vi "IDN.vi"(8 "error in (no error)":errorcluster, 9 "Low module address":i32=120, 10 "High module address":i32=123, 11 "RP Communicator in":refnum<class "RP Communicator.lvclass">) -> (0 "error out":errorcluster, 1 "Logic tag":u16, 2 "IDN response":u32=1 format="0x%x (%d)", 3 "RP Communicator out":refnum<class "RP Communicator.lvclass">, 4 "Status response":u32=1 format="0x%x (%d)", 5 "DDS modulus":i64, 6 "Module":i32)   [LabVIEW 2024, in "RP Communicator.lvclass"]
uses:
  RP Communicator.lvclass
  RP Communicator.lvclass/RP Communicator.ctl
  RP Command.ctl
  RP Write Command TCP.vi
  RP Read Status TCP.vi
  RP Status Offsets.ctl
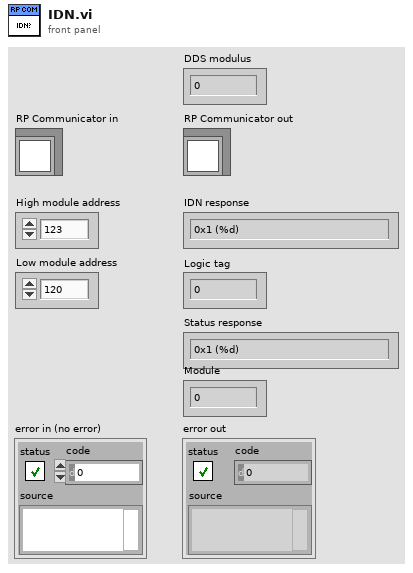
[diagram p1: front panel]
types:
  T1 = typedef "RP Command.ctl" = enum16{"Reset", "Read IDN", "Stop server", "Get status", "Get temperature", "Connect client", "Arm", "Software trigger", "Get whole buffer", "Get chunk", "System call", "Get config", "Set config", "Recieve data", "Recieve Calibartion", "Transmit data"}
  T2 = enum16{"big-endian, network order", "native, host order", "little-endian"}
  T3 = typedef "RP Status Offsets.ctl" = u16
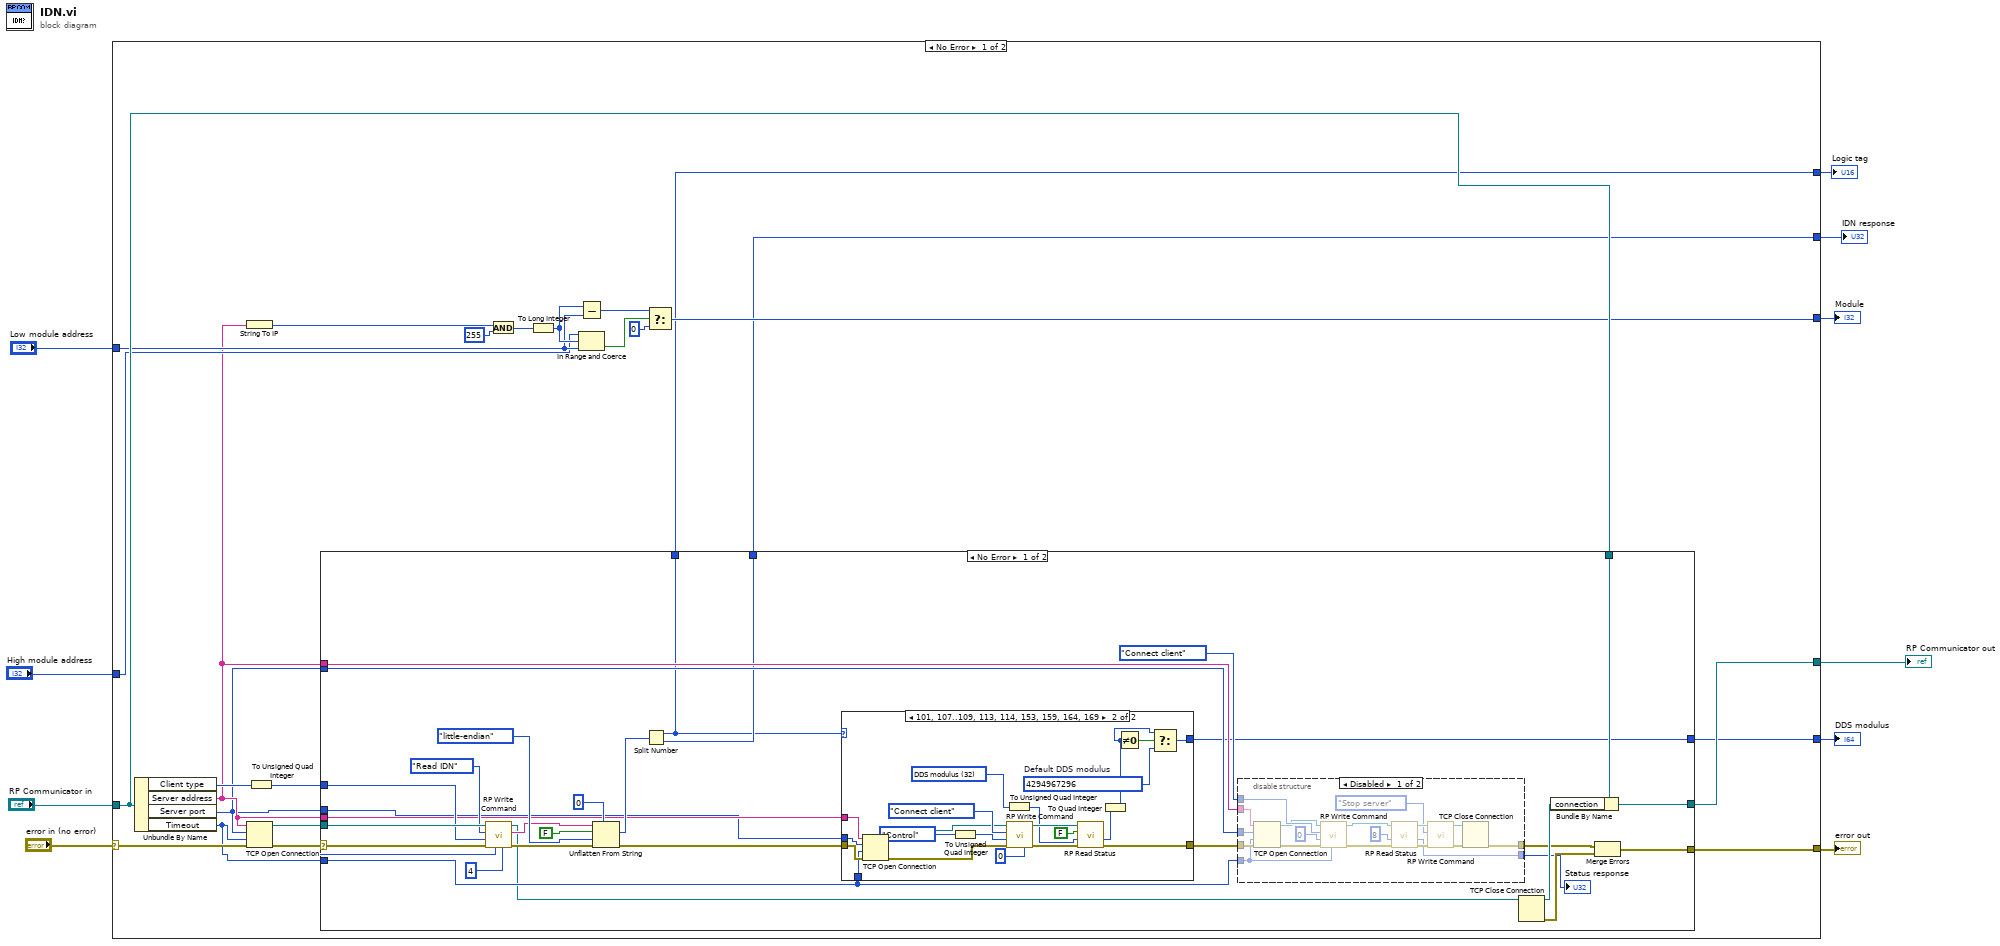
[diagram p0: block diagram]
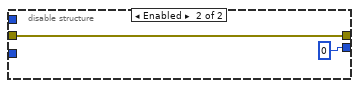
[diagram p3: hidden frame]
diagram:
  n1 = case shown="No Error" "error in (no error)" {
    selector: "error in (no error)" -> [w34 w110]
    tunnel: [w28 w110] -> w9
    tunnel: [w30 w109] -> w7
    tunnel: "RP Communicator in" -> [w31 w109]
    tunnel: [w17 _] -> w6
    tunnel: "Low module address" -> [w22 _]
    tunnel: "High module address" -> [w21 _]
    tunnel: [w16 _] -> w3
    tunnel: [w15 _] -> w2
    tunnel: [w14 _] -> w1
    frame No Error {
      n2 = Unbundle By Name(w31) -> ("Client type"=w32:enum16{"Control", "Reciever", "Transmitter"}, "Server address"=w12:string, "Server port"=w11:u16, "Timeout"=w27:i32)
      n3 = String To IP(1:w12) -> (0:w26:u32)
      n4 = TCP Open Connection(address=w12, remote port or service name=w11, timeout ms (60000)=w27, error in (no error)=w34) -> (connection ID=w33:refnum<k5>, error out=w13:errorcluster)  [unwired: 1 in]
      n5 = To Unsigned Quad Integer(1:w32) -> (0:w29:u64)
      n6 = case shown="No Error" w13 {
        selector: w13 -> [w39 w108]
        tunnel: w33 -> [w64 _]
        tunnel: w31 -> [w63 w107]
        tunnel: [w62 w107] -> w30
        tunnel: w29 -> [w60 _]
        tunnel: [w54 w108] -> w28
        tunnel: w11 -> [w50 _]
        tunnel: w27 -> [w36 _]
        tunnel: w12 -> [w48 _]
        tunnel: [w45 _] -> w16
        tunnel: [w41 _] -> w15
        tunnel: [w40 _] -> w14
        tunnel: w12 -> [w38 _]
        tunnel: w11 -> [w37 _]
        frame No Error {
          n7 = call-poly "RP Write Command.vi"("bytes to read"=4, "timeout ms (25000)"=w36, "Error In"=w39, "Command payload"=w60, "Command number"=RP_Command."Read IDN", "connection ID"=w64) -> ("Error Out"=w44:errorcluster, "data out"=w46:string, "connection ID out"=w35:refnum<k5>)  [unwired: 2 in, 1 out]
          n8 = Unflatten From String(type=u32 0, binary string=w46, data includes array or string size? (T)=FALSE, byte order (0:big-endian, network order)=T2."little-endian", error in (no error)=w44) -> (value=w56:u32, error out=w43:errorcluster)  [unwired: 1 out]
          n9 = Split Number(x=w56) -> (hi(x)=w40:u16, lo(x)=w41:u16)
          n10 = case shown="101, 107..109, 113, 114, 153, 159, 164, 169" w40 {
            tunnel: [_ w75] -> w45
            tunnel: w43 -> [w65 w72]
            tunnel: [w65 w74] -> w42
            tunnel: w38 -> [_ w70]
            tunnel: w37 -> [_ w69]
            tunnel: w36 -> [_ w68]
            frame 0, Default {
            }
            frame 101, 107..109, 113, 114, 153, 159, 164, 169 {
              w78 = i64 4294967296  # Default DDS modulus
              w82 = T3 32 items=["Writer address"=0, "Record start position"=4, "Trig state and ID"=8, "Phase"=12, "X1"=16, "Y1"=20, "RxFIFO counter or  X2"=24, "TxFIFO counter or Y2"=28, "DDS modulus"=32] ("Status offsets")
              n11 = TCP Open Connection(address=w70, remote port or service name=w69, timeout ms (60000)=w68, error in (no error)=w72) -> (connection ID=w67:refnum<k5>, error out=w71:errorcluster)  [unwired: 1 in]
              n12 = To Unsigned Quad Integer(1:enum16{"Control", "Reciever", "Transmitter"}."Control" ("Client type")) -> (0:w84:u64)
              n13 = To Unsigned Quad Integer(1:w82) -> (0:w81:u64)
              n14 = call-poly "RP Write Command.vi"("bytes to read"=0, "Error In"=w71, "Command payload"=w84, "Command number"=RP_Command."Connect client", "connection ID"=w67) -> ("Error Out"=w80:errorcluster, "connection ID out"=w83:refnum<k5>)  [unwired: 3 in, 2 out]
              n15 = call-poly "RP Read Status.vi"("Error In"=w80, "Status offset"=w81, "Read config"=FALSE, "connection ID"=w83) -> ("Error Out"=w74:errorcluster, "Status response"=w76:u32)  [unwired: 5 in, 1 out]
              n16 = To Quad Integer(1:w76) -> (0:w73:i64)
              n17 = Not Equal To 0?(x=w73) -> (x != 0?=w77:bool)
              n18 = Select(t=w73, s=w77, f=w78) -> (s? t:f=w75:i64)
            }
          }
          n19 = disable-structure shown="Disabled" {
            disable-tunnel: w42 -> [w103 w106]
            disable-tunnel: [w91 w106] -> w52
            disable-tunnel: RP_Command."Connect client" ("Command number") -> [w101 _]
            disable-tunnel: w48 -> [w99 _]
            disable-tunnel: w50 -> [w98 _]
            disable-tunnel: w36 -> [w97 _]
            disable-tunnel: [w87 u32 0 ("Status response")] -> w49
            frame Disabled {
              n20 = TCP Open Connection(address=w99, remote port or service name=w98, timeout ms (60000)=w97, error in (no error)=w103) -> (connection ID=w100:refnum<k5>, error out=w102:errorcluster)  [unwired: 1 in]
              n21 = call-poly "RP Write Command.vi"("timeout ms (25000)"=w97, "Error In"=w102, "Command payload"=u64 0, "Command number"=w101, "connection ID"=w100) -> ("Error Out"=w94:errorcluster, "connection ID out"=w95:refnum<k5>)  [unwired: 3 in, 2 out]
              n22 = call-poly "RP Read Status.vi"("Error In"=w94, "Status offset"=u64 8, "connection ID"=w95) -> ("Error Out"=w93:errorcluster, "Status response"=w87:u32, "connection ID out"=w89:refnum<k5>)  [unwired: 6 in]
              n23 = call-poly "RP Write Command.vi"("Error In"=w93, "Command number"=RP_Command."Stop server", "connection ID"=w89) -> ("Error Out"=w92:errorcluster, "connection ID out"=w90:refnum<k5>)  [unwired: 5 in, 2 out]
              n24 = TCP Close Connection(connection ID=w90, error in (no error)=w92) -> (error out=w91:errorcluster)  [unwired: 1 in, 1 out]
            }
            frame Enabled {
            }
          }
          "Status response" <- w49
          n25 = TCP Close Connection(connection ID=w35) -> (connection ID out=w55:refnum<k5>, error out=w53:errorcluster)  [unwired: 2 in]
          n26 = Bundle By Name(cluster=w63, "connection"=w55) -> (w62:refnum<class "RP Communicator.lvclass">)
          n27 = Merge Errors(w52, w53) -> (w54:errorcluster)
        }
        frame Error {
        }
      }
      n28 = And(x=w26, y=u32 255) -> (x .and. y?=w24:u32)
      n29 = To Long Integer(number=w24) -> (32bit integer=w23:i32)
      n30 = Subtract(x=w23, y=w22) -> (x-y=w18:i32)
      n31 = In Range and Coerce(upper limit=w21, x=w23, lower limit=w22) -> (In Range?=w20:bool)  [unwired: 1 out]
      n32 = Select(t=w18, s=w20, f=0) -> (s? t:f=w17:i32)
    }
    frame Error {
    }
  }
  "error out" <- w9
  "RP Communicator out" <- w7
  "Module" <- w6
  "DDS modulus" <- w3
  "IDN response" <- w2
  "Logic tag" <- w1
